vi "Drive.vi"(8 "Backward?":bool, 9 "Distance":dbl, 11 "Boolean in":bool) -> (3 "Boolean out":bool)   [LabVIEW 2014]
uses:
  Support Files/Global Data!!!.vi
  <vilib>/addons/control/pid/pid.llb/PID (DBL).vi
  <vilib>/addons/control/pid/NI_PID_pid.lvlib
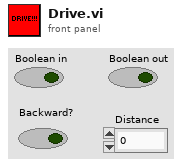
[diagram p1: front panel]
types:
  T1 = cluster{"proportional gain (Kc)":dbl, "integral time (Ti, min)":dbl, "derivative time (Td, min)":dbl}
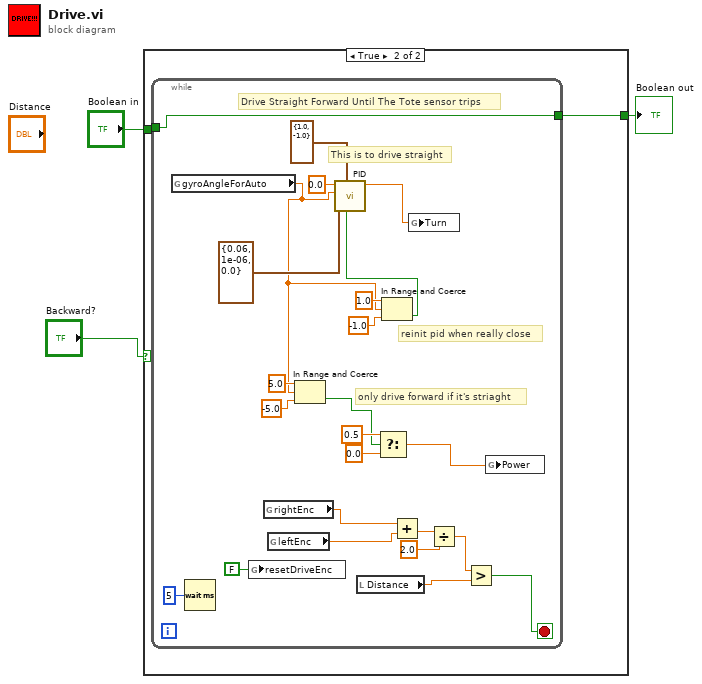
[diagram p0: block diagram]
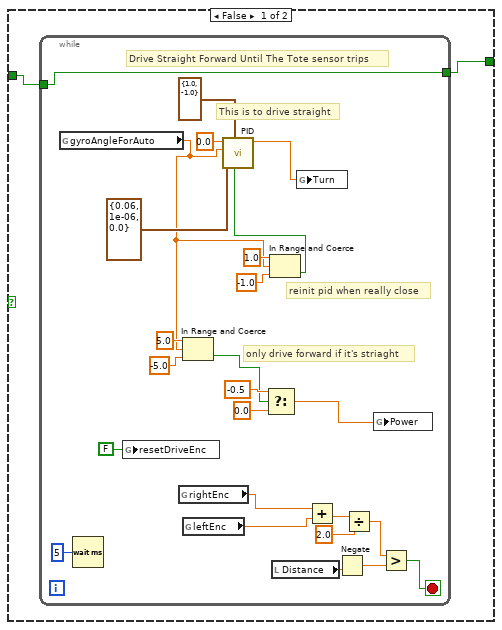
[diagram p2: hidden frame]
diagram:
  n1 = case shown="True" "Backward?" {
    tunnel: "Boolean in" -> [w5 w32]
    tunnel: [w4 w31] -> w2
    frame False {
      n2 = while {
        tunnel: [w15] -> w4
        tunnel: w5 -> [w15]
        stop <- w7 stop-if-true
        # "reinit pid when really close"
        # "Drive Straight Forward Until The Tote sensor trips"
        # "only drive forward if it's striaght"
        # "This is to drive straight"
        n3 = global read "Global Data!!!.vi" "gyroAngleForAuto"() -> (w17:dbl)
        n4 = Wait (ms)(milliseconds to wait=u32 5) -> ()  [unwired: 1 out]
        n5 = global write "Global Data!!!.vi" "resetDriveEnc"(FALSE ("resetDriveEnc")) -> ()
        n6 = global read "Global Data!!!.vi" "rightEnc"() -> (w13:dbl)
        n7 = In Range and Coerce(upper limit=5.0, x=w17, lower limit=-5.0) -> (In Range?=w20:bool)  [unwired: 1 out]
        n8 = global read "Global Data!!!.vi" "leftEnc"() -> (w12:dbl)
        n9 = Select(t=-0.5, s=w20, f=0.0) -> (s? t:f=w26:dbl)
        n10 = In Range and Coerce(upper limit=1.0, x=w17, lower limit=-1.0) -> (In Range?=w16:bool)  [unwired: 1 out]
        n11 = call-poly <vilib>:"PID.vi"("reinitialize? (F)"=w16, "output range"=cluster{"output high":dbl, "output low":dbl} {"output high"=1.0, "output low"=-1.0}, "PID gains"=T1 {"proportional gain (Kc)"=0.06, "integral time (Ti, min)"=1e-06, "derivative time (Td, min)"=0.0}, "process variable"=w17, "setpoint"=0.0) -> ("output"=w29:dbl)  [unwired: 5 in, 1 out]
        n12 = local read "Distance"() -> (w8:dbl)
        n13 = global write "Global Data!!!.vi" "Turn"(w29) -> ()
        n14 = Add(x=w13, y=w12) -> (x+y=w11:dbl)
        n15 = Negate(x=w8) -> (-x=w6:dbl)
        n16 = Divide(x=w11, y=2.0) -> (x/y=w9:dbl)
        n17 = global write "Global Data!!!.vi" "Power"(w26) -> ()
        n18 = Greater?(x=w9, y=w6) -> (0:w7:bool)
      }
    }
    frame True {
      n19 = while {
        tunnel: [w41] -> w31
        tunnel: w32 -> [w41]
        stop <- w34 stop-if-true
        # "reinit pid when really close"
        # "Drive Straight Forward Until The Tote sensor trips"
        # "only drive forward if it's striaght"
        # "This is to drive straight"
        n20 = global read "Global Data!!!.vi" "gyroAngleForAuto"() -> (w43:dbl)
        n21 = Wait (ms)(milliseconds to wait=u32 5) -> ()  [unwired: 1 out]
        n22 = global write "Global Data!!!.vi" "resetDriveEnc"(FALSE ("resetDriveEnc")) -> ()
        n23 = global read "Global Data!!!.vi" "rightEnc"() -> (w39:dbl)
        n24 = global read "Global Data!!!.vi" "leftEnc"() -> (w38:dbl)
        n25 = In Range and Coerce(upper limit=5.0, x=w43, lower limit=-5.0) -> (In Range?=w46:bool)  [unwired: 1 out]
        n26 = local read "Distance"() -> (w33:dbl)
        n27 = Select(t=0.5, s=w46, f=0.0) -> (s? t:f=w52:dbl)
        n28 = In Range and Coerce(upper limit=1.0, x=w43, lower limit=-1.0) -> (In Range?=w42:bool)  [unwired: 1 out]
        n29 = call-poly <vilib>:"PID.vi"("reinitialize? (F)"=w42, "output range"=cluster{"output high":dbl, "output low":dbl} {"output high"=1.0, "output low"=-1.0}, "PID gains"=T1 {"proportional gain (Kc)"=0.06, "integral time (Ti, min)"=1e-06, "derivative time (Td, min)"=0.0}, "process variable"=w43, "setpoint"=0.0) -> ("output"=w55:dbl)  [unwired: 5 in, 1 out]
        n30 = Add(x=w39, y=w38) -> (x+y=w37:dbl)
        n31 = global write "Global Data!!!.vi" "Turn"(w55) -> ()
        n32 = Divide(x=w37, y=2.0) -> (x/y=w35:dbl)
        n33 = Greater?(x=w35, y=w33) -> (0:w34:bool)
        n34 = global write "Global Data!!!.vi" "Power"(w52) -> ()
      }
    }
  }
  "Boolean out" <- w2
